vi "Convert Variant To DBL.vi"(10 "error in (no error)":errorcluster, 11 "Variant":variant) -> (2 "error out":errorcluster, 3 "DBL":dbl)   [LabVIEW 2020, in "RTAF.lvlib"]
uses:
  RTAF.lvlib
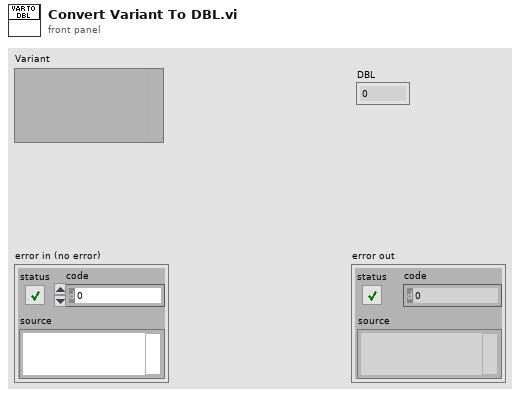
[diagram p1: front panel]
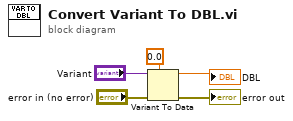
[diagram p0: block diagram]
diagram:
  n1 = Variant To Data(error in="error in (no error)", type=0.0, Variant="Variant") -> (data=→"DBL":dbl, error out=→"error out":errorcluster)
